vi "Write Frame.vi"(8 "error in (no error)":errorcluster, 10 "ARGB Image in":T1, 11 "Writer (Greyscale) in":refnum<class "Writer (Greyscale).lvclass">) -> (0 "error out":errorcluster, 3 "Writer (Greyscale)":refnum<class "Writer (Greyscale).lvclass">)   [LabVIEW 2020, in "video_io.lvlib" / "Writer (Greyscale).lvclass"]
uses:
  Writer (Greyscale).lvclass
  Writer (Greyscale).lvclass/Writer (Greyscale).ctl
  0e3f49b0-4303-46d3-b8ab-944fedc4b55e.vi
  image/Greyscale Image.ctl
  image/image.lvlib
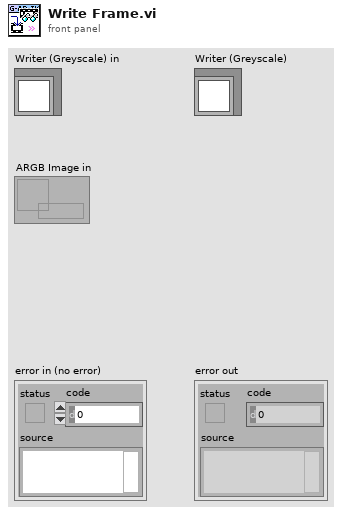
[diagram p1: front panel]
types:
  T1 = typedef "image.lvlib/Greyscale Image.ctl" = refnum<data-value>
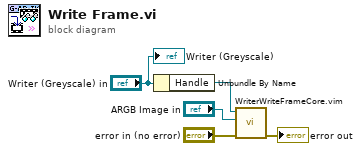
[diagram p0: block diagram]
diagram:
  n1 = Unbundle By Name("Writer (Greyscale) in") -> ("Handle"=w4:refnum<data-value>)
  n2 = call "WriterWriteFrameCore.vim"("error in (no error)"="error in (no error)", "Greyscale Image"="ARGB Image in", "Handle"=w4) -> ("error out"=→"error out":errorcluster)  [unwired: 8 in]
  "Writer (Greyscale)" <- "Writer (Greyscale) in"
